vi "Compile Engine Init - Multi FPGA.vi"(8 "error in (no error)":errorcluster, 11 "Device Item Ref in":T2 format="%.0x") -> (0 "error out":errorcluster, 2 "System":T1, 3 "Device Item Ref out":T2 format="%.0x")   [LabVIEW 2015, in "Engine Simulation Toolkit System Explorer.lvlib"]
uses:
  Engine Simulation Toolkit System Explorer.lvlib
  <vilib>/NI Veristand/Custom Device API/Custom Device Item Ref.ctl
  Shared/Engine Init Data.ctl
  <vilib>/NI Veristand/Custom Device API/Custom Device Channel Type.ctl
  Shared/Properties.vi
  <vilib>/NI Veristand/Custom Device API/Get Item Property (I32).vi
  <vilib>/NI Veristand/Custom Device API/Get Item Property (String).vi
  Shared/Engine Simulation Toolkit Shared.lvlib
  <vilib>/NI Veristand/Custom Device API/Custom Device API.lvlib
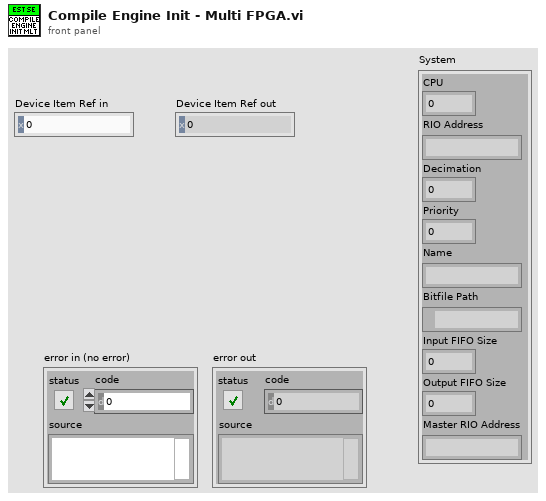
[diagram p1: front panel]
types:
  T1 = typedef "Engine Simulation Toolkit Shared.lvlib/Engine Init Data.ctl" = cluster{"CPU":i32, "RIO Address":string, "Decimation":i64, "Priority":i32, "Name":string, "Bitfile Path":path, "Input FIFO Size":i32, "Output FIFO Size":i32, "Master RIO Address":string}
  T2 = typedef "Custom Device API.lvlib/Custom Device Item Ref.ctl" = u64
  T3 = typedef "Custom Device API.lvlib/Custom Device Channel Type.ctl" = enum16{"Input", "Output"}
  T4 = typedef "Custom Device API.lvlib/Custom Device Timed Loop Priority.ctl" = enum32{"Low", "Medium", "High"}
  T5 = typedef "Custom Device API.lvlib/Custom Device Item Info.ctl" = cluster{"Name":string, "Is Channel":bool, "GUID":string, "Is Waveform":bool}
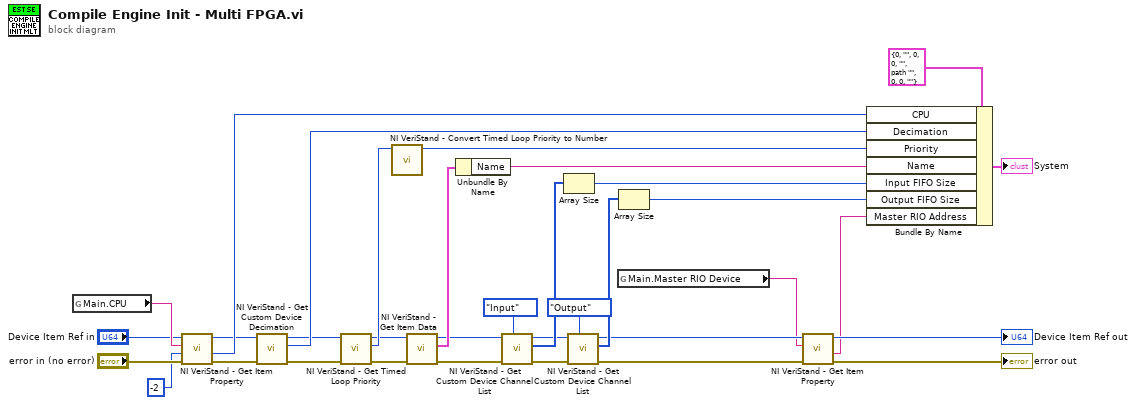
[diagram p0: block diagram]
diagram:
  n1 = global read "Properties.vi" "Main.CPU"() -> (w32:string)
  n2 = call-poly <vilib>:"NI VeriStand - Get Item Property.vi"("error in (no error)"="error in (no error)", "Default Value"=-2, "Property Name"=w32, "Item Ref in"="Device Item Ref in") -> ("error out"=w28:errorcluster, "Value"=w30:i32, "Item Ref out"=w29:T2)  [unwired: 4 in, 1 out]
  n3 = call <vilib>:"NI VeriStand - Get Custom Device Decimation.vi"("error in (no error)"=w28, "Device Ref in"=w29) -> ("error out"=w27:errorcluster, "Decimation"=w26:i32, "Device Ref out"=w24:T2)  [unwired: 7 in]
  n4 = call <vilib>:"NI VeriStand - Get Timed Loop Priority.vi"("error in (no error)"=w27, "Device Ref in"=w24) -> ("error out"=w25:errorcluster, "Priority"=w23:T4, "Device Ref out"=w21:T2)  [unwired: 7 in]
  n5 = call <vilib>:"NI VeriStand - Convert Timed Loop Priority to Number.vi"("Priority"=w23) -> ("Numeric Priority"=w22:i32)  [unwired: 10 in]
  n6 = call <vilib>:"NI VeriStand - Get Item Data.vi"("error in (no error)"=w25, "Item Ref in"=w21) -> ("error out"=w17:errorcluster, "Item Info"=w20:T5, "Item Ref out"=w16:T2)  [unwired: 6 in, 1 out]
  n7 = Unbundle By Name(w20) -> ("Name"=w7:string)
  n8 = call <vilib>:"NI VeriStand - Get Custom Device Channel List.vi"("Channel Type"=Custom_Device_Channel_Type."Input", "error in (no error)"=w17, "Device Ref in"=w16) -> ("error out"=w15:errorcluster, "Specified Channel Ref List"=w13:T2[], "Device Ref out"=w11:T2)  [unwired: 6 in]
  n9 = Array Size(array=w13) -> (size(s)=w12:i32)
  n10 = call <vilib>:"NI VeriStand - Get Custom Device Channel List.vi"("Channel Type"=Custom_Device_Channel_Type."Output", "error in (no error)"=w15, "Device Ref in"=w11) -> ("error out"=w5:errorcluster, "Specified Channel Ref List"=w9:T2[], "Device Ref out"=w6:T2)  [unwired: 6 in]
  n11 = global read "Properties.vi" "Main.Master RIO Device"() -> (w1:string)
  n12 = Array Size(array=w9) -> (size(s)=w8:i32)
  n13 = call-poly <vilib>:"NI VeriStand - Get Item Property.vi"("error in (no error)"=w5, "Property Name"=w1, "Item Ref in"=w6) -> ("error out"=→"error out":errorcluster, "Value"=w2:string, "Item Ref out"=→"Device Item Ref out":T2)  [unwired: 5 in, 1 out]
  n14 = Bundle By Name(cluster=T1 {"CPU"=0, "RIO Address"="", "Decimation"=0, "Priority"=0, "Name"="", "Bitfile Path"=path "", "Input FIFO Size"=0, "Output FIFO Size"=0, "Master RIO Address"=""} ("System"), "CPU"=w30, "Decimation"=w26, "Priority"=w22, "Name"=w7, "Input FIFO Size"=w12, "Output FIFO Size"=w8, "Master RIO Address"=w2) -> (→"System":T1)
